vi "Updater Get Spartan Database Path.vi"(6 "DEBUG? (f)":bool, 8 "error in (no error)":errorcluster, 11 "Spartan Install Path (empty)":path) -> (0 "error out":errorcluster, 3 "Spartan Database Path":path)   [LabVIEW 2011]
uses:
  <vilib>/Utility/config.llb/Read Key (Path).vi
  <vilib>/Utility/config.llb/NI_LVConfig.lvlib
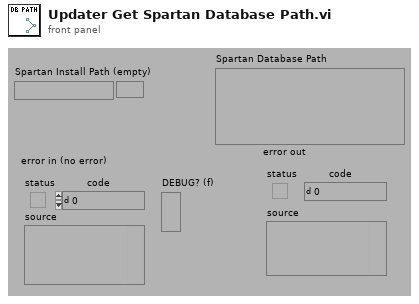
[diagram p1: front panel]
types:
  T1 = typedef "NI_LVConfig.lvlib/Config Data RefNum.ctl" = refnum<k1>
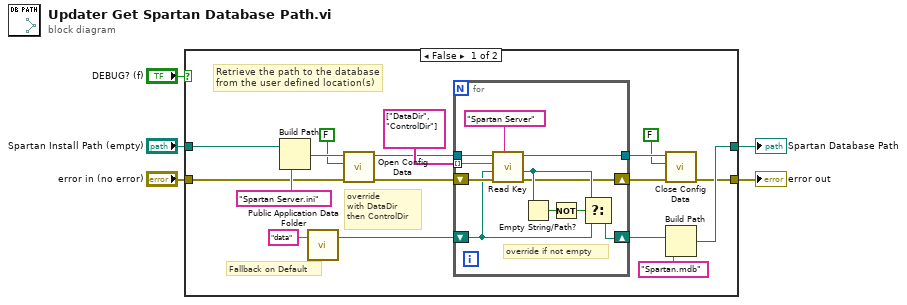
[diagram p0: block diagram]
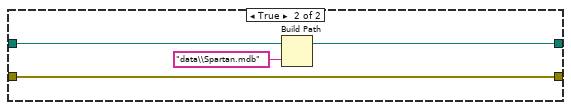
[diagram p2: hidden frame]
diagram:
  n1 = case shown="False" "DEBUG? (f)" {
    tunnel: [w18 w34] -> w5
    tunnel: "Spartan Install Path (empty)" -> [w8 w35]
    tunnel: "error in (no error)" -> [w17 w37]
    tunnel: [w16 w37] -> w2
    frame False {
      # "Retrieve the path to the database\nfrom the user defined location(s)"
      # "override \nwith DataDir\nthen ControlDir"
      # "Fallback on Default"
      n2 = Build Path(base path=w8, name or relative path="Spartan Server.ini") -> (appended path=w21:path)
      n3 = call "Public Application Data Folder.vi"("Relative Path (\"\" - Folder)"="data" ("name or relative path")) -> ("Client Storage Path"=w6:path)  [unwired: 2 in]
      n4 = call <vilib>:"Open Config Data.vi"("error in (no error)"=w17, "create file if necessary (T)"=FALSE, "configuration file path"=w21) -> ("error out"=w14:errorcluster, "refnum"=w13:T1)  [unwired: 6 in, 1 out]
      n5 = for {
        tunnel: string[] ["DataDir", "ControlDir"] -> [w30] mode=indexing
        shift-right: [w26] -> w11
        shift-left: w14 -> [w27]
        tunnel: w13 -> [w29]
        tunnel: [w28] -> w12
        shift-right: [w24] -> w10
        shift-left: w6 -> [w25]
        # "override if not empty"
        n6 = call-poly <vilib>:"Read Key.vi"("section"="Spartan Server" ("directive name"), "error in (no error)"=w27, "default value"=w25, "key"=w30, "refnum"=w29) -> ("error out"=w26:errorcluster, "value"=w31:path, "refnum out"=w28:T1)  [unwired: 4 out]
        n7 = Empty String/Path?(string/path=w31) -> (empty?=w33:bool)
        n8 = Not(x=w33) -> (.not. x?=w32:bool)
        n9 = Select(t=w31, s=w32, f=w25) -> (s? t:f=w24:path)
      }
      n10 = call <vilib>:"Close Config Data.vi"("error in (no error)"=w11, "write file if changed (T)"=FALSE, "refnum"=w12) -> ("error out"=w16:errorcluster)  [unwired: 8 out]
      n11 = Build Path(base path=w10, name or relative path="Spartan.mdb") -> (appended path=w18:path)
    }
    frame True {
      n12 = Build Path(base path=w35, name or relative path="data\\Spartan.mdb") -> (appended path=w34:path)
    }
  }
  "Spartan Database Path" <- w5
  "error out" <- w2
